vi "DAQmx Read (Counter U32 1Chan 1Samp).vi"(0 "task/channels in":refnum<k21>, 9 "timeout":dbl=10.0 format="%0.2f", 11 "error in":errorcluster) -> (4 "task out":refnum<k21>, 6 "data":u32, 15 "error out":errorcluster)   [LabVIEW 2013]
doc: "Reads a 32-bit unsigned integer sample from a counter task. Use an instance that reads 32-bit unsigned integers when NI-DAQmx returns counter samples unscaled, such as for event counting."
uses:
  nilvaiu.dll
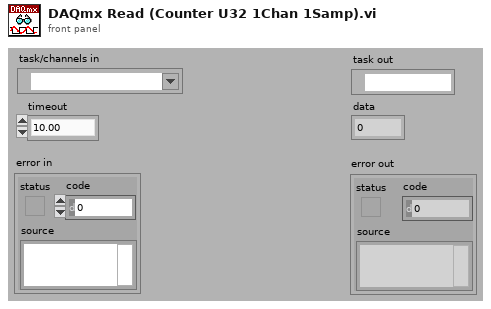
[diagram p1: front panel]
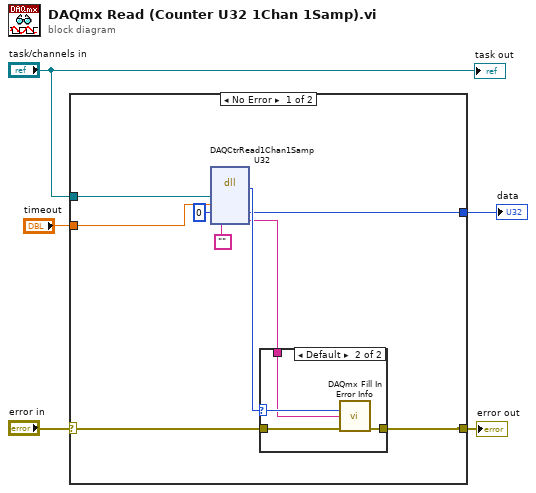
[diagram p0: block diagram]
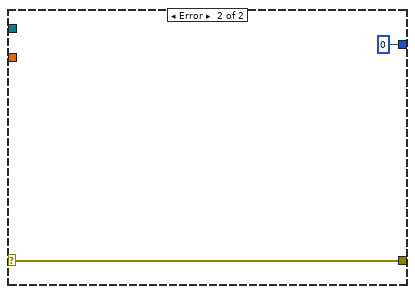
[diagram p3: hidden frame]
diagram:
  n1 = case shown="No Error" "error in" {
    selector: "error in" -> [w7 w20]
    tunnel: [w13 w20] -> w4
    tunnel: "task/channels in" -> [w14 _]
    tunnel: [w8 u32 0 ("data")] -> w2
    tunnel: "timeout" -> [w6 _]
    frame No Error {
      n2 = dll-call lib="nilvaiu.*" fn="DAQCtrRead1Chan1SampU32"("taskID"=w14, "timeout"=w6, "data"=u32 0, "extendedErrorInfo"="") -> (w12:i32, "data"=w8:u32, "extendedErrorInfo"=w9:string)  [unwired: 4 in, 3 out]
      n3 = case shown="Default" w12 {
        selector: w12 -> [_ w17]
        tunnel: w7 -> [w15 w19]
        tunnel: [w15 w18] -> w13
        tunnel: w9 -> [_ w16]
        frame 0 {
        }
        frame Default {
          n4 = call "DAQmx Fill In Error Info.vi"("status code"=w17, "extended error info"=w16, "error in"=w19) -> ("error out"=w18:errorcluster)  [unwired: 1 in, 11 out]
        }
      }
    }
    frame Error {
    }
  }
  "error out" <- w4
  "data" <- w2
  "task out" <- "task/channels in"
